vi "set_params.vi"(8 "error in (no error)":errorcluster caption="entrée d'erreur (pas d'erreur)", 11 "MiniBatchSparsePCA.lvclass 2":refnum<class "MiniBatchSparsePCA.lvclass">) -> (0 "error out":errorcluster caption="sortie d'erreur", 3 "MiniBatchSparsePCA.lvclass":refnum<class "MiniBatchSparsePCA.lvclass">)   [LabVIEW 2020, in "MiniBatchSparsePCA.lvclass"]
uses:
  MiniBatchSparsePCA.lvclass
  MiniBatchSparsePCA.lvclass/MiniBatchSparsePCA.ctl
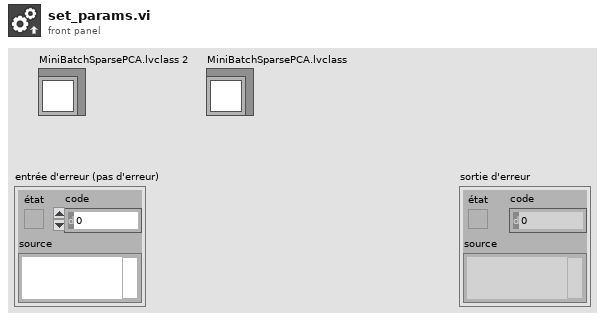
[diagram p1: front panel]
types:
  T1 = typedef "mini_batch_sparse_pca_params.ctl" = cluster{"n_components":cluster{"n_components_type":string, "n_components_int":dbl}, "alpha":dbl, "ridge_alpha":dbl, "n_iter":dbl, "batch_size":dbl, "verbose":dbl, "shuffle":bool, "n_jobs":dbl, "method":string, "random_state":dbl}
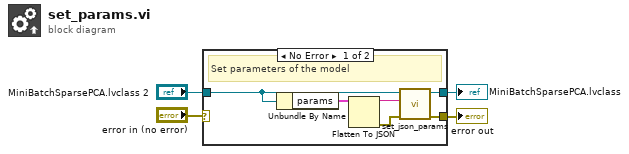
[diagram p0: block diagram]
diagram:
  n1 = case shown="No Error" "error in (no error)" {
    selector: "error in (no error)" -> [_ w12]
    tunnel: [w7 w12] -> w3
    tunnel: [w8 w11] -> w1
    tunnel: "MiniBatchSparsePCA.lvclass 2" -> [w5 w11]
    frame No Error {
      # "Set parameters of the model"
      n2 = Unbundle By Name(w5) -> ("params"=w10:T1)
      n3 = Flatten To JSON(anything=w10) -> (JSON string=w9:string, 11:w6:errorcluster)  [unwired: 2 in]
      n4 = call-dynamic "set_json_params.vi"("error in (no error)"=w6, "params"=w9, "Model en entrée"=w5) -> ("error out"=w7:errorcluster, "Model en sortie"=w8:refnum<class "MiniBatchSparsePCA.lvclass">)  [unwired: 7 in]
    }
    frame Error {
    }
  }
  "error out" <- w3
  "MiniBatchSparsePCA.lvclass" <- w1
